vi "CalculatePhaseSensitivity.vi"(2 "delta L":dbl, 3 "n":i32, 4 "L":dbl) -> (1 "Czułość fazowa":dbl)   [LabVIEW 2014]
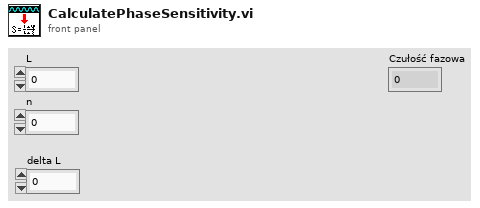
[diagram p1: front panel]
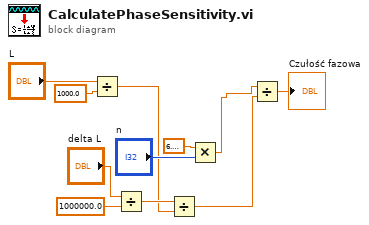
[diagram p0: block diagram]
diagram:
  n1 = Divide(x="L", y=1000.0) -> (x/y=w1:dbl)
  n2 = Divide(x="delta L", y=1000000.0) -> (x/y=w2:dbl)
  n3 = Divide(x=w2, y=w1) -> (x/y=w4:dbl)
  n4 = Multiply(x=6.283185307179586, y="n") -> (x*y=w3:dbl)
  n5 = Divide(x=w3, y=w4) -> (x/y=→"Czułość fazowa":dbl)
